vi "Can_SendIgn.vi"(9 "Interface:Baud Rate":u32=250000, 10 "cluster (:memory:)":refnum<k21>="Z177TEST", 11 "interface":refnum<k21>="CAN2") -> ()   [LabVIEW 2015]
uses:
  Crl/Can_DataType.ctl
  <vilib>/xnet/xnet.llb/XNET Frame CAN.ctl
  <vilib>/xnet/xnet.llb/XNET Frame Type CAN.ctl
  <vilib>/xnet/xnet.llb/XNET Create Session (Frame Output Stream).vi
  <vilib>/xnet/xnet.llb/XNET Write (Frame CAN).vi
  <resource>/objmgr/xnet.rc
panel:
  in  "error in (no error)":errorcluster
  in  "IGN":T1=[{"identifier"=1046, "payload"=[253, 24, 191, 255, 255, 255, 255, 255], "Send?"=TRUE, "Note"="点火1", "Delays"=200, "Seq"=0}, {"identifier"=749, "payload"=[240, 15, 0, 0, 0, 0, 0, 0], "Send?"=TRUE, "Note"="点火2", "Delays"=200, "Seq"=0}, {"identifier"=415, "payload"=[0, 0, 120, 0, 0, 0, 0, 0], "Send?"=TRUE, "Note"="点火3", "Delays"=200, "Seq"=0}] {"payload" format="%02x"; "identifier" format="%x"}
  # "ms"
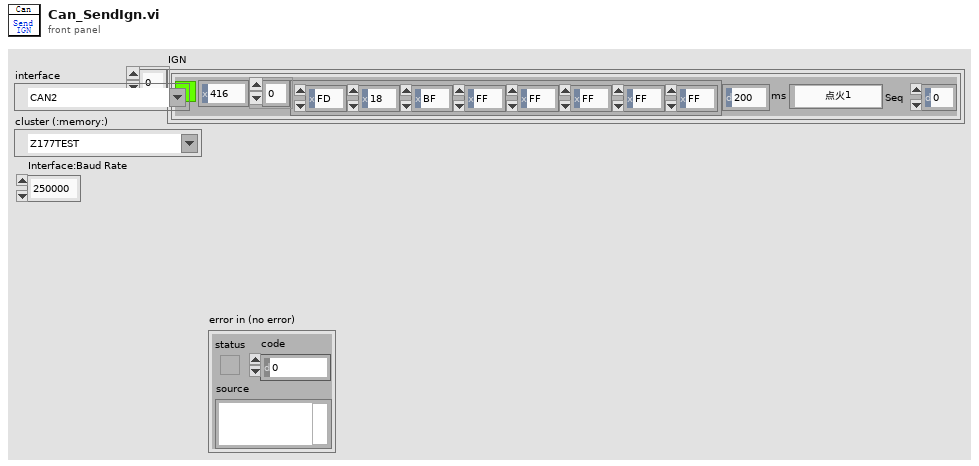
[diagram p1: front panel]
types:
  T1 = typedef "Can_DataType.ctl" = cluster{"identifier":u32, "payload":u8[], "Send?":bool, "Note":string, "Delays":u32, "Seq":i32}[]
  T2 = typedef "XNET Frame CAN.ctl" = cluster{"timestamp":timestamp, "payload":u8[], "identifier":u32, "type":T3, "extended?":bool, "echo?":bool}
  T3 = typedef "XNET Frame Type CAN.ctl" = u8
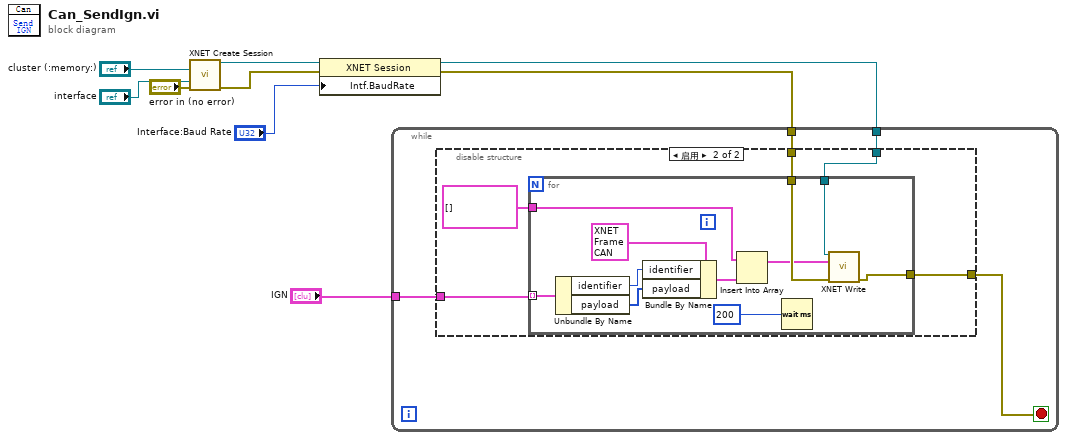
[diagram p0: block diagram]
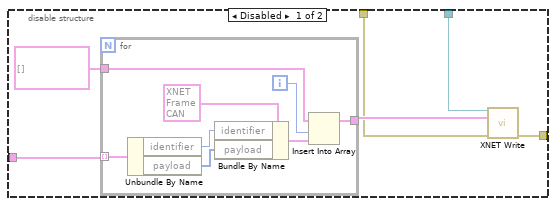
[diagram p2: hidden frame]
diagram:
  n1 = call-poly <vilib>:"XNET Create Session.vi"("cluster (:memory:)"="cluster (:memory:)", "interface"="interface", "error in (no error)"="error in (no error)") -> ("session out"=w7:refnum<k21>, "error out"=w9:errorcluster)  [unwired: 11 out]
  n2 = property class="XNET Session"(reference=w7, error in=w9, "Intf.BaudRate"="Interface:Baud Rate") -> (reference out=w2:refnum<k21>, error out=w3:errorcluster)
  n3 = while {
    tunnel: w3 -> [w13]
    tunnel: w2 -> [w12]
    tunnel: "IGN" -> [w10]
    stop <- w11 stop-if-true
    n4 = disable-structure shown="启用" {
      disable-tunnel: w13 -> [w17 w30]
      disable-tunnel: w12 -> [w16 w29]
      disable-tunnel: [w15 w28] -> w11
      disable-tunnel: w10 -> [w14 w31]
      frame Disabled {
        n5 = for {
          tunnel: w14 -> [w20] mode=indexing
          tunnel: T2[] [] ("data") -> [w25]
          tunnel: [w21] -> w18
          i -> [w24]
          n6 = Unbundle By Name(w20) -> ("identifier"=w26:u32, "payload"=w27:u8[])
          n7 = Bundle By Name(cluster=T2 {"timestamp"=timestamp(0 s since 1904-01-01), "payload"=[], "identifier"=0, "type"=0, "extended?"=FALSE, "echo?"=FALSE} ("CAN frame"), "identifier"=w26, "payload"=w27) -> (w22:T2)
          n8 = Insert Into Array(array=w25, index=w24, new element=w22) -> (w21:T2[])
        }
        n9 = call-poly <vilib>:"XNET Write.vi"("session in"=w16, "data"=w18, "error in (no error)"=w17) -> ("error out"=w15:errorcluster)  [unwired: 12 out]
      }
      frame Enabled {
        n10 = for {
          tunnel: w31 -> [w38] mode=indexing
          tunnel: T2[] [] ("data") -> [w41]
          tunnel: w30 -> [w37]
          tunnel: w29 -> [w36]
          tunnel: [w34] -> w28
          n11 = Unbundle By Name(w38) -> ("identifier"=w42:u32, "payload"=w43:u8[])
          n12 = Bundle By Name(cluster=T2 {"timestamp"=timestamp(0 s since 1904-01-01), "payload"=[], "identifier"=0, "type"=0, "extended?"=FALSE, "echo?"=FALSE} ("CAN frame"), "identifier"=w42, "payload"=w43) -> (w39:T2)
          n13 = Insert Into Array(array=w41, new element=w39) -> (w35:T2[])  [unwired: 1 in]
          n14 = Wait (ms)(milliseconds to wait=u32 200 ("等待时间（毫秒）")) -> ()  [unwired: 1 out]
          n15 = call-poly <vilib>:"XNET Write.vi"("session in"=w36, "data"=w35, "error in (no error)"=w37) -> ("error out"=w34:errorcluster)  [unwired: 12 out]
        }
      }
    }
  }
